vi "Main.vi"(10 "Sub Panel":refnum<vi>, 11 "Module Admin":refnum<class "Delacor_lib_QMH_Module Admin.lvclass">) -> ()   [LabVIEW 2019, in "ANALISIS .lvlib"]
doc: "This template is based off of the Queued Message Handler design pattern and the Queued Message Handler project template that ships with LabVIEW.\n\nThe main difference is that the queue is private to this module and communication between modules is performed via Broadcast and Request events.\n\nRequest events are wrapped in public API methods and are handled in the Event Handling Loop (EHL) of this VI. Any module can register for Broadcast events sent by this module. The EHL generates messages based on user interface actions.\n\nThe Message Handling Loop (MHL) processes messages generated by the EHL, or by other messages. The messages are string values, so new messages can be added easily to the Message Cases case structure in the MHL. Each message cluster can also provide an optional value for Message Data, which is a variant that can be converted to whatever message-specific data is required.\n_____\nBased on Delacor QMH Project Template 5.0.0.82."
uses:
  ANALISIS .lvlib
  <vilib>/Delacor/Delacor QMH/Libraries/Module Admin_class/Delacor_lib_QMH_Module Admin.lvclass
  Module Data--cluster.ctl
  STOP HELPER LOOP ANALISIS Argument--cluster.ctl
  <vilib>/Delacor/Delacor QMH/Libraries/Message Queue_class/Delacor_lib_QMH_Message Queue.lvclass/Delacor_lib_QMH_Message Queue.ctl
  Stop Argument--cluster.ctl
  <vilib>/Delacor/Delacor QMH/Libraries/Module Admin_class/Delacor_lib_QMH_Module Admin.lvclass/Delacor_lib_QMH_Module Admin.ctl
  START HELPER LOOP ANALISIS Argument--cluster.ctl
  acq datos recibir Argument--cluster.ctl
  <vilib>/Utility/miscctls.llb/LVPointTypeDef.ctl
  <vilib>/Delacor/Delacor QMH/Libraries/Message Queue_class/Delacor_lib_QMH_Enqueue Message (Single).vi
  <vilib>/Delacor/Delacor QMH/Libraries/Module Admin_class/Delacor_lib_QMH_Get External Launch.vi
  <vilib>/Utility/error.llb/Error Cluster From Error Code.vi
  <vilib>/ErrorRing/Error Ring.xnode
  <vilib>/Delacor/Delacor QMH/Libraries/Message Queue_class/Delacor_lib_QMH_Message Queue.lvclass
panel:
  out "Bomba encendida":bool
  out "Alarma":bool
  out "Porcentaje del tanque":dbl
  out "Tanque":dbl(slide) scale=0.0..100.0
  out "Estado del tanque":string
  out "Velocidad de bomba de llenado":dbl(knob) scale=0.0..100.0
  out "Velocidad de la bomba de llenado":dbl
  in  "Simulate MHL Error":bool
  in  "Simulate EHL Error":bool
  out "error out":errorcluster
  out "Status":string
  # "Alarmas"
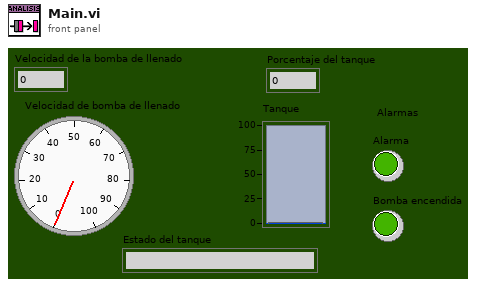
[diagram p1: front panel]
types:
  T1 = typedef "ANALISIS .lvlib/Request Events--cluster.ctl" = cluster{"Stop Module":refnum<user-event>, "Show Panel":refnum<user-event>, "Hide Panel":refnum<user-event>, "Get Module Execution Status":refnum<user-event>, "Show Diagram":refnum<user-event>, "START HELPER LOOP ANALISIS":refnum<user-event>, "STOP HELPER LOOP ANALISIS":refnum<user-event>, "acq datos recibir":refnum<user-event>}
  T2 = typedef "ANALISIS .lvlib/Module Data--cluster.ctl" = cluster{"Status":string}
  T3 = typedef "ANALISIS .lvlib/STOP HELPER LOOP ANALISIS Argument--cluster.ctl" = cluster{"Boolean":bool}
  T4 = enum32{"invalid lock state", "Not Locked", "Locked (No Password)", "Password-protected"}
  T5 = typedef "ANALISIS .lvlib/Stop Argument--cluster.ctl" = cluster{"Origin":string, "Exit via Stop Module Req?":bool, "Wait for Module to stop?":bool}
  T6 = typedef "ANALISIS .lvlib/START HELPER LOOP ANALISIS Argument--cluster.ctl" = cluster{"DELAY TIMEOUT":i32}
  T7 = typedef "ANALISIS .lvlib/acq datos recibir Argument--cluster.ctl" = cluster{"Numeric":dbl}
  T8 = typedef "LVPointTypeDef.ctl" = cluster{"Horizontal":i16, "Vertical":i16}
  T9 = enum32{"Invalid", "Standard", "Closed", "Hidden", "Minimized", "Maximized"}
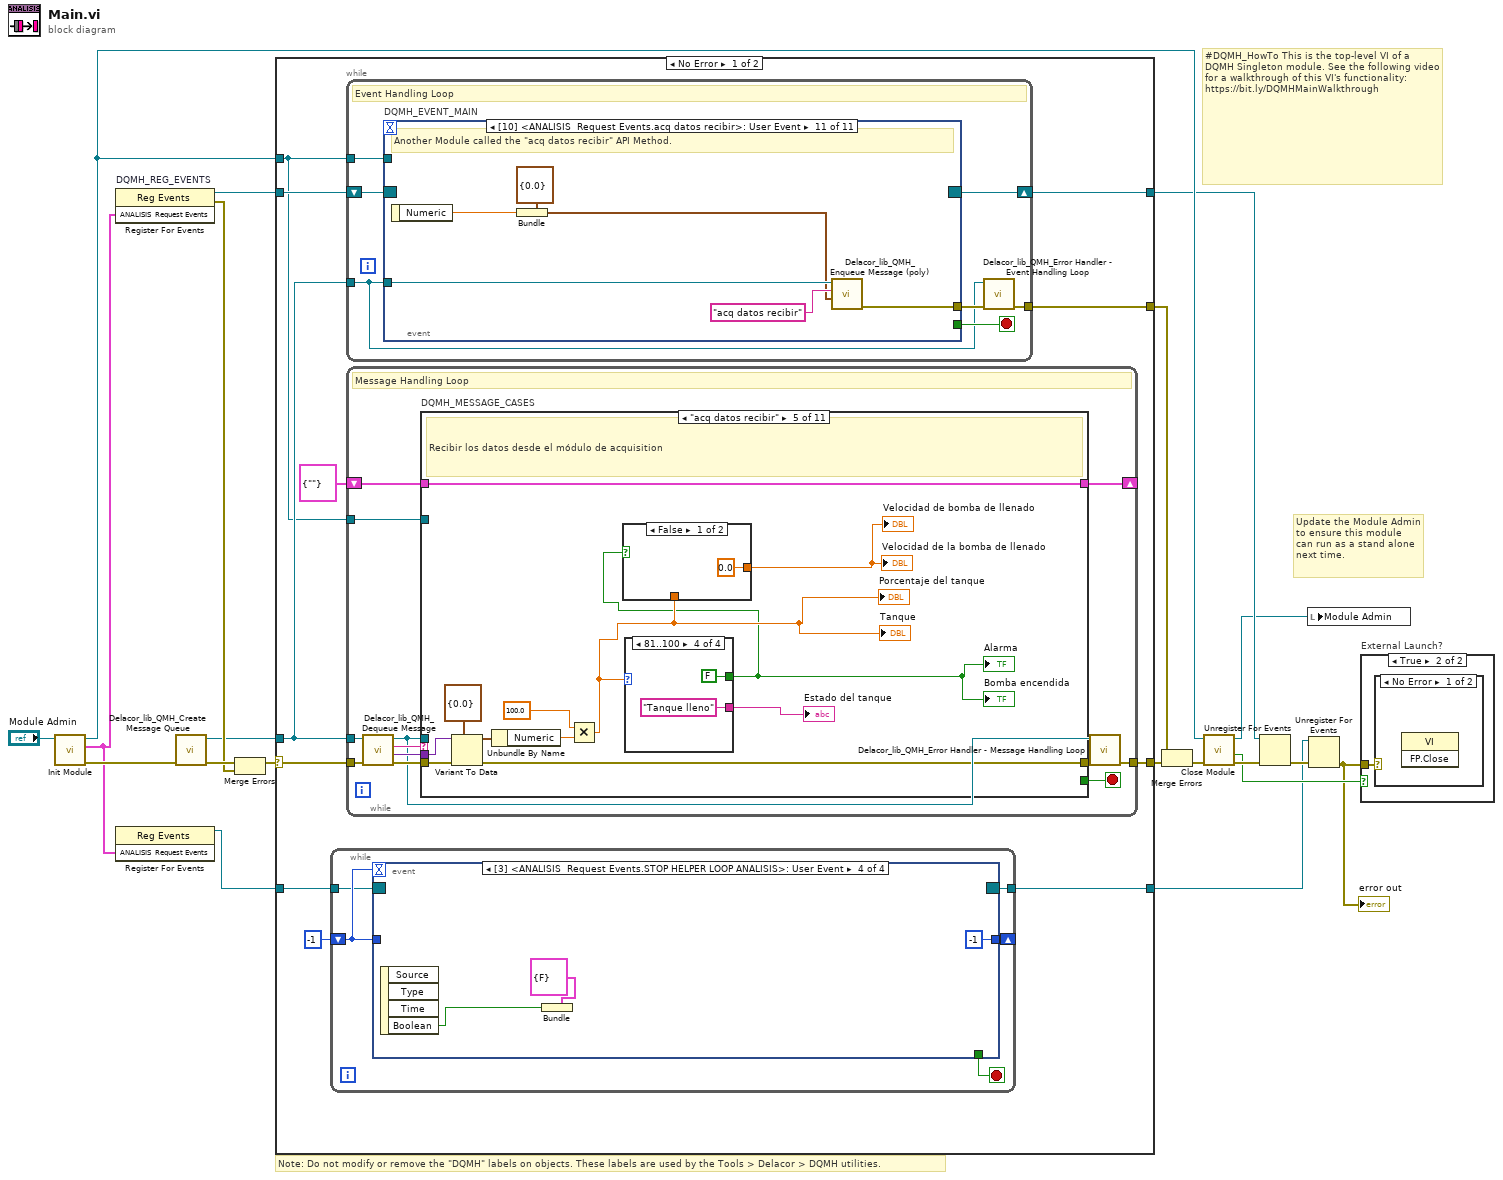
[diagram p0: block diagram]
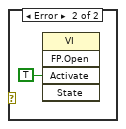
[diagram p3: hidden frame]
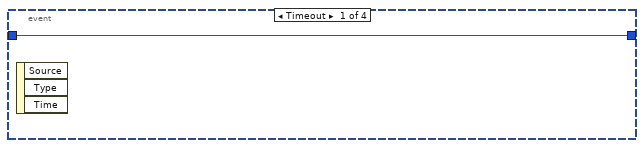
[diagram p4: hidden frame]
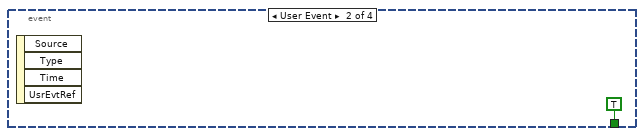
[diagram p5: hidden frame]
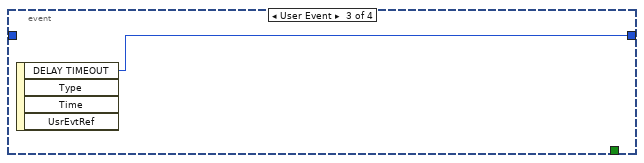
[diagram p6: hidden frame]
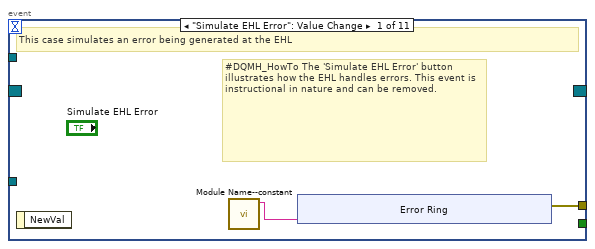
[diagram p7: hidden frame]
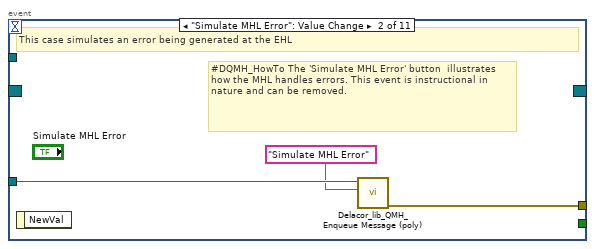
[diagram p8: hidden frame]
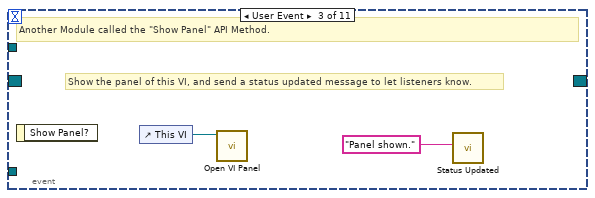
[diagram p9: hidden frame]
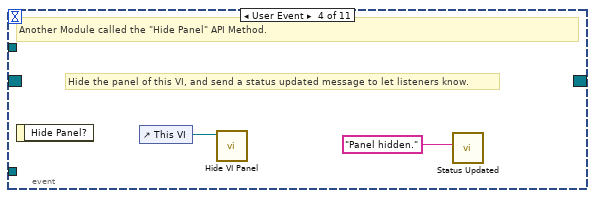
[diagram p10: hidden frame]
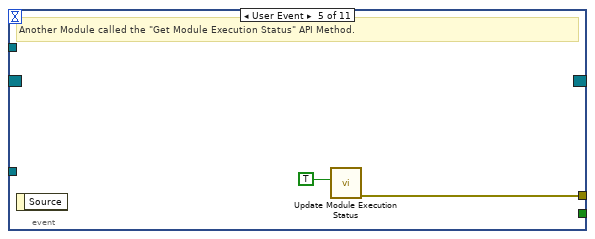
[diagram p11: hidden frame]
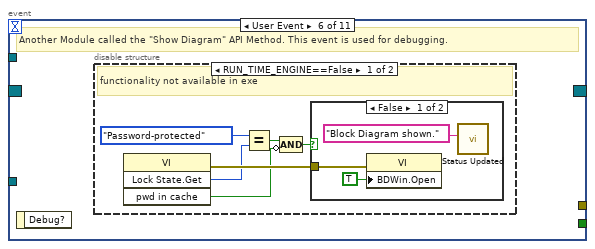
[diagram p12: hidden frame]
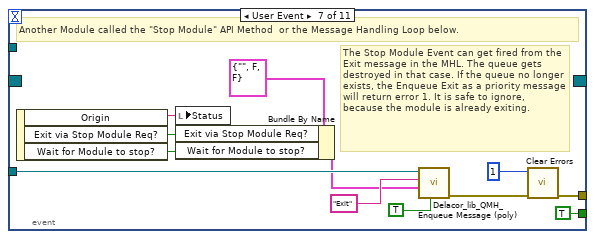
[diagram p15: hidden frame]
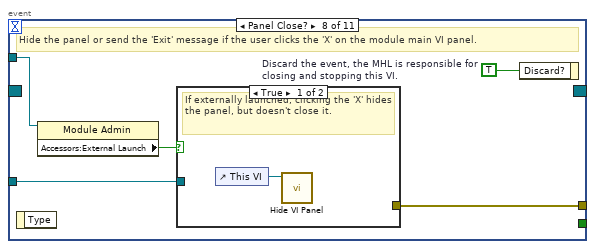
[diagram p16: hidden frame]
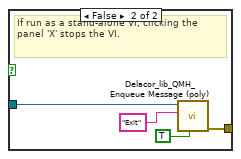
[diagram p17: hidden frame]
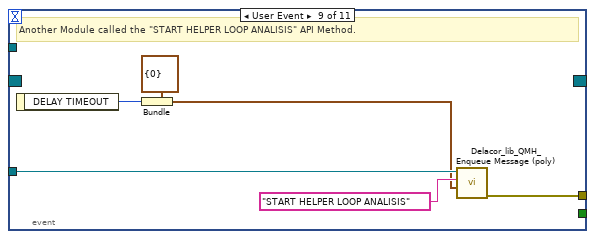
[diagram p18: hidden frame]
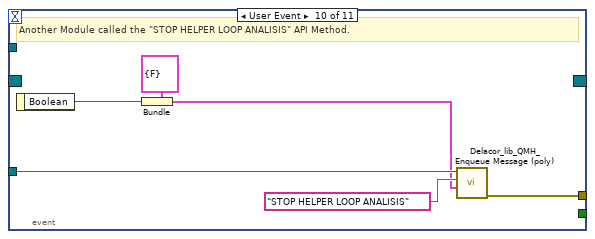
[diagram p19: hidden frame]
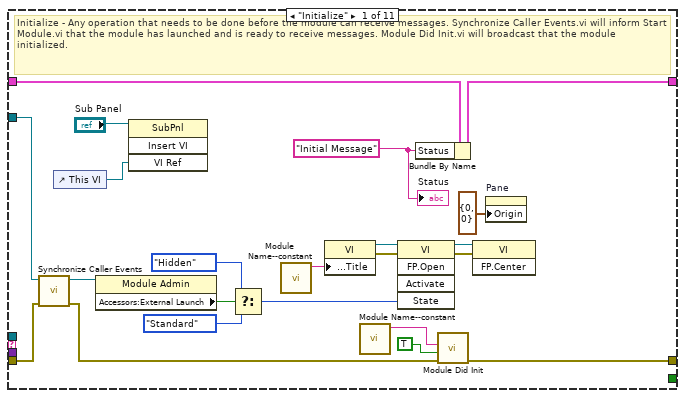
[diagram p20: hidden frame]
diagram:
  # "#DQMH_HowTo This is the top-level VI of a DQMH Singleton module. See the following video for a walkthrough of this VI's functionality: https://bit.ly/DQMHMainWalkthrough"
  # "Note: Do not modify or remove the \"DQMH\" labels on objects. These labels are used by the Tools > Delacor > DQMH utilities."
  # "Update the Module Admin to ensure this module can run as a stand alone next time."
  n1 = call "Init Module.vi"("Singleton Module Admin in"="Module Admin") -> ("error out"=w19:errorcluster, "ANALISIS  Request Events"=w5:T1, "Singleton Module Admin out"=w12:refnum<class "Delacor_lib_QMH_Module Admin.lvclass">)  [unwired: 8 in]
  n2 = register-events "DQMH_REG_EVENTS"(w5) -> (reference out=w10:refnum<event-registration>, error out=w13:errorcluster)  [unwired: 2 in]
  n3 = register-events(w5) -> (reference out=w4:refnum<event-registration>)  [unwired: 2 in, 1 out]
  n4 = call <vilib>:"Delacor_lib_QMH_Create Message Queue.vi"("error in (no error)"=w19) -> ("error out"=w15:errorcluster, "Message Queue"=w9:refnum<class "Delacor_lib_QMH_Message Queue.lvclass">)  [unwired: 9 in]
  n5 = Merge Errors(w15, w13) -> (w14:errorcluster)
  n6 = case shown="No Error" w14 {
    selector: w14 -> [w29 w255]
    tunnel: [w31 w254] -> w20
    tunnel: [w28 w260] -> w11
    tunnel: w10 -> [w26 w260]
    tunnel: w9 -> [w25 w253]
    tunnel: [w30 _] -> w17
    tunnel: w12 -> [w24 w256]
    tunnel: w4 -> [w22 w252]
    tunnel: [w21 w252] -> w2
    frame No Error {
      n7 = while {
        tunnel: [w36] -> w21
        shift-right: [w34] -> _
        shift-left: -1 ("DELAY TIMEOUT") -> [w33]
        tunnel: w22 -> [w32]
        stop <- w35 stop-if-true
        n8 = event shown="[3] <ANALISIS  Request Events.STOP HELPER LOOP ANALISIS>: User Event" {
          selector: w32 -> [_ _ _ _]
          dyn-events: [_ _ _ _] -> w36
          timeout: w33 -> [_ _ _ _]
          tunnel: [_ TRUE ("stop") _ _] -> w35
          tunnel: [w37 _ w39 -1 ("DELAY TIMEOUT")] -> w34
          tunnel: w33 -> [w37 _ _ _]
          event Timeout {
            n9 = event-data() -> ()  [unwired: 1 in, 3 out]
          }
          event User Event {
            n10 = event-data() -> ()  [unwired: 1 in, 4 out]
          }
          event User Event {
            n11 = event-data() -> ("DELAY TIMEOUT"=w39:i32)  [unwired: 1 in, 3 out]
          }
          event User Event {
            n12 = event-data() -> ("Boolean"=w41:bool)  [unwired: 1 in, 3 out]
            n13 = Bundle(cluster=T3 {"Boolean"=FALSE} ("STOP HELPER LOOP ANALISIS Argument"), "Boolean"=w41) -> ()  [unwired: 1 out]
          }
        }
      }
      n14 = while {
        tunnel: w25 -> [w43]
        shift-right: [w46] -> w28
        shift-left: w26 -> [w47]
        tunnel: [w48] -> w30
        tunnel: w24 -> [w44]
        stop <- w45 stop-if-true
        # "Event Handling Loop"
        n15 = event "DQMH_EVENT_MAIN" shown="[10] <ANALISIS  Request Events.acq datos recibir>: User Event" {
          selector: w47 -> [_ _ _ _ _ _ _ _ _ _ _]
          dyn-events: [_ _ _ _ _ _ _ _ _ _ _] -> w46
          timeout: _ -> [_ _ _ _ _ _ _ _ _ _ _]
          tunnel: [_ _ _ _ _ _ TRUE ("Discard?") _ _ _ _] -> w45
          tunnel: w43 -> [_ w60 _ _ _ _ w84 w91 w104 w110 w116]
          tunnel: [w51 w61 _ _ w67 _ w87 w93 w99 w105 w111] -> w49
          tunnel: w44 -> [_ _ _ _ _ _ _ w90 _ _ _]
          event "Simulate EHL Error": Value Change {
            # "#DQMH_HowTo The 'Simulate EHL Error' button  illustrates how the EHL handles errors. This event is instructional in nature and can be removed."
            # "This case simulates an error being generated at the EHL"
            n16 = event-data() -> ()  [unwired: 1 in, 1 out]
            n17 = call "Module Name--constant.vi"() -> ("Module Name"=w50:string)  [unwired: 11 in]
            n18 = xnode "Error Ring"("parameter 0"=w50) -> ("error out"=w51:errorcluster)
          }
          event "Simulate MHL Error": Value Change {
            # "#DQMH_HowTo The 'Simulate MHL Error' button  illustrates how the MHL handles errors. This event is instructional in nature and can be removed."
            # "This case simulates an error being generated at the EHL"
            n19 = event-data() -> ()  [unwired: 1 in, 1 out]
            n20 = call-poly <vilib>:"Delacor_lib_QMH_Enqueue Message (poly).vi"("Message"="Simulate MHL Error", "Message Queue in"=w60) -> ("error out"=w61:errorcluster)  [unwired: 8 in, 1 out]
          }
          event User Event {
            # "Show the panel of this VI, and send a status updated message to let listeners know."
            # "Another Module called the \"Show Panel\" API Method."
            n21 = event-data() -> ()  [unwired: 1 in, 1 out]
            n22 = control-ref of="This VI"() -> (w63:refnum<vi>)
            n23 = call "Open VI Panel.vi"("VI"=w63) -> ()  [unwired: 10 in, 1 out]
            n24 = call "Status Updated.vi"("Status"="Panel shown." ("format string")) -> ()  [unwired: 10 in, 1 out]
          }
          event User Event {
            # "Hide the panel of this VI, and send a status updated message to let listeners know."
            # "Another Module called the \"Hide Panel\" API Method."
            n25 = event-data() -> ()  [unwired: 1 in, 1 out]
            n26 = control-ref of="This VI"() -> (w65:refnum<vi>)
            n27 = call "Hide VI Panel.vi"("VI"=w65) -> ()  [unwired: 10 in, 1 out]
            n28 = call "Status Updated.vi"("Status"="Panel hidden." ("format string")) -> ()  [unwired: 10 in, 1 out]
          }
          event User Event {
            # "Another Module called the \"Get Module Execution Status\" API Method."
            n29 = event-data() -> ()  [unwired: 1 in, 1 out]
            n30 = call "Update Module Execution Status.vi"("Running?"=TRUE) -> ("error out"=w67:errorcluster)  [unwired: 10 in]
          }
          event User Event {
            # "Another Module called the \"Show Diagram\" API Method. This event is used for debugging."
            n31 = event-data() -> ()  [unwired: 1 in, 1 out]
            n32 = disable-structure shown="RUN_TIME_ENGINE==False" {
              frame condition #0 (active) {
                # "functionality not available in exe"
                n33 = invoke class="VI" method="Lock State.Get"() -> (error out=w73:errorcluster, "Get Lock State"=w72:T4, "pwd in cache"=w69:bool)  [unwired: 4 in, 1 out]
                n34 = Equal?(x=T4."Password-protected", y=w72) -> (x = y?=w70:bool)
                n35 = Compound Arithmetic op=AND(w70, invert w69) -> (w68:bool)
                n36 = case shown="False" w68 {
                  tunnel: w73 -> [w76 _]
                  frame False {
                    n37 = property class="VI"(error in=w76, "BDWin.Open"=TRUE ("Block Diagram Window:Open")) -> ()  [unwired: 1 in, 2 out]
                    n38 = call "Status Updated.vi"("Status"="Block Diagram shown." ("format string")) -> ()  [unwired: 10 in, 1 out]
                  }
                  frame True {
                    # "Password-protected VI, and the password is not in the cache. Do not show the diagram."
                  }
                }
              }
              frame condition #1 {
              }
            }
          }
          event User Event {
            # "The Stop Module Event can get fired from the Exit message in the MHL. The queue gets destroyed in that case. If the queue no longer exists, the Enqueue Exit as a priority message will return error 1. It is safe to ignore, because the module is already exiting."
            # "Another Module called the \"Stop Module\" API Method  or the Message Handling Loop below."
            n39 = event-data() -> ("Origin"=w83:string, "Exit via Stop Module Req?"=w79:bool, "Wait for Module to stop?"=w78:bool)  [unwired: 1 in]
            n40 = local write "Status"(w83) -> ()
            n41 = Bundle By Name(cluster=T5 {"Origin"="", "Exit via Stop Module Req?"=FALSE, "Wait for Module to stop?"=FALSE} ("Stop Argument"), "Exit via Stop Module Req?"=w79, "Wait for Module to stop?"=w78) -> (w77:T5)
            n42 = call-poly <vilib>:"Delacor_lib_QMH_Enqueue Message (poly).vi"("Priority Message? (F)"=TRUE, "Message Data"=w77, "Message"="Exit", "Message Queue in"=w84) -> ("error out"=w88:errorcluster)  [unwired: 6 in, 1 out]
            n43 = call <vilib>:"Clear Errors.vi"("error in (no error)"=w88, "specific error code to clear (0: all)"=1) -> ("error out"=w87:errorcluster)  [unwired: 4 in, 1 out]
          }
          event Panel Close? {
            w92 = TRUE  # Discard the event, the MHL is responsible for closing and stopping this VI.
            # "Hide the panel or send the 'Exit' message if the user clicks the 'X' on the module main VI panel."
            n44 = event-data() -> ()  [unwired: 1 in, 1 out]
            n45 = property class="Module Admin"(reference=w90) -> ("Accessors:External Launch"=w89:bool)  [unwired: 1 in, 2 out]
            n46 = case shown="True" w89 {
              tunnel: w91 -> [_ w97]
              tunnel: [_ w98] -> w93
              frame True {
                # "If externally launched, clicking the 'X' hides the panel, but doesn't close it."
                n47 = control-ref of="This VI"() -> (w94:refnum<vi>)
                n48 = call "Hide VI Panel.vi"("VI"=w94) -> ()  [unwired: 10 in, 1 out]
              }
              frame False {
                # "If run as a stand-alone VI, clicking the panel 'X' stops the VI."
                n49 = call-poly <vilib>:"Delacor_lib_QMH_Enqueue Message (poly).vi"("Priority Message? (F)"=TRUE, "Message"="Exit", "Message Queue in"=w97) -> ("error out"=w98:errorcluster)  [unwired: 7 in, 1 out]
              }
            }
            n50 = event-data("Discard?"=w92) -> ()  [unwired: 1 in, 1 out]
          }
          event User Event {
            # "Another Module called the \"START HELPER LOOP ANALISIS\" API Method."
            n51 = event-data() -> ("DELAY TIMEOUT"=w100:i32)  [unwired: 1 in]
            n52 = Bundle(cluster=T6 {"DELAY TIMEOUT"=0} ("START HELPER LOOP ANALISIS Argument"), "DELAY TIMEOUT"=w100) -> (w101:T6)
            n53 = call-poly <vilib>:"Delacor_lib_QMH_Enqueue Message (poly).vi"("Message Data"=w101, "Message"="START HELPER LOOP ANALISIS", "Message Queue in"=w104) -> ("error out"=w99:errorcluster)  [unwired: 7 in, 1 out]
          }
          event User Event {
            # "Another Module called the \"STOP HELPER LOOP ANALISIS\" API Method."
            n54 = event-data() -> ("Boolean"=w106:bool)  [unwired: 1 in]
            n55 = Bundle(cluster=T3 {"Boolean"=FALSE} ("STOP HELPER LOOP ANALISIS Argument"), "Boolean"=w106) -> (w107:T3)
            n56 = call-poly <vilib>:"Delacor_lib_QMH_Enqueue Message (poly).vi"("Message Data"=w107, "Message"="STOP HELPER LOOP ANALISIS", "Message Queue in"=w110) -> ("error out"=w105:errorcluster)  [unwired: 7 in, 1 out]
          }
          event User Event {
            # "Another Module called the \"acq datos recibir\" API Method."
            n57 = event-data() -> ("Numeric"=w112:dbl)  [unwired: 1 in]
            n58 = Bundle(cluster=T7 {"Numeric"=0.0} ("acq datos recibir Argument"), "Numeric"=w112) -> (w113:T7)
            n59 = call-poly <vilib>:"Delacor_lib_QMH_Enqueue Message (poly).vi"("Message Data"=w113, "Message"="acq datos recibir", "Message Queue in"=w116) -> ("error out"=w111:errorcluster)  [unwired: 7 in, 1 out]
          }
        }
        n60 = call-dynamic "Delacor_lib_QMH_Error Handler - Event Handling Loop.vi"("error in (no error)"=w49, "Message Queue in"=w43) -> ("dup error in"=w48:errorcluster)  [unwired: 8 in, 1 out]
      }
      n61 = while {
        tunnel: w25 -> [w119]
        shift-right: [w123] -> _
        shift-left: T2 {"Status"=""} ("Data Cluster") -> [w124]
        tunnel: w29 -> [w127]
        tunnel: [w125] -> w31
        tunnel: w24 -> [w117]
        stop <- w122 stop-if-true
        # "Message Handling Loop"
        n62 = call-dynamic "Delacor_lib_QMH_Dequeue Message.vi"("error in (no error)"=w127, "Message Queue in"=w119) -> ("error out"=w126:errorcluster, "Message Data"=w120:variant, "Message"=w121:string, "Message Queue out"=w118:refnum<class "Delacor_lib_QMH_Message Queue.lvclass">)  [unwired: 6 in]
        n63 = case "DQMH_MESSAGE_CASES" shown="\"acq datos recibir\"" w121 {
          selector: w121 -> [_ _ _ _ _ _ _ _ _ _ w239]
          tunnel: w118 -> [_ _ _ _ _ _ _ _ w209 w231 _]
          tunnel: w126 -> [w148 w152 w158 w164 w176 w191 w193 w198 w216 w237 w241]
          tunnel: [w146 w152 w156 w162 w174 w190 w193 w197 w212 w234 w242] -> w128
          tunnel: w124 -> [w137 w151 w157 w163 w175 w189 w192 w195 w211 w230 w240]
          tunnel: [w136 w151 w157 w163 w175 w189 w192 w195 w211 w230 w240] -> w123
          tunnel: [_ _ _ _ _ _ _ _ _ w229 _] -> w122
          tunnel: w120 -> [_ _ w155 w161 w173 _ _ _ w210 w228 _]
          tunnel: w117 -> [w138 _ _ _ _ _ _ _ w208 w223 _]
          frame "Initialize" {
            w131 = "Initial Message" ("Initial Message")
            # "Initialize - Any operation that needs to be done before the module can receive messages. Synchronize Caller Events.vi will inform Start Module.vi that the module has launched and is ready to receive messages. Module Did Init.vi will broadcast that the module initialized."
            n64 = call "Synchronize Caller Events.vi"("error in (no error)"=w148, "Singleton Module Admin in"=w138) -> ("error out"=w147:errorcluster, "Singleton Module Admin out"=w133:refnum<class "Delacor_lib_QMH_Module Admin.lvclass">)  [unwired: 8 in]
            n65 = control-ref of="This VI"() -> (w129:refnum<vi>)
            n66 = property class="Module Admin"(reference=w133) -> ("Accessors:External Launch"=w142:bool)  [unwired: 1 in, 2 out]
            n67 = invoke class="SubPnl" method="Insert VI"(reference="Sub Panel", "VI Ref"=w129) -> ()  [unwired: 2 in, 4 out]
            n68 = Select(t=T9."Hidden" ("State"), s=w142, f=T9."Standard" ("State")) -> (s? t:f=w139:T9)
            n69 = call "Module Name--constant.vi"() -> ("Module Name"=w145:string)  [unwired: 11 in]
            n70 = property class="VI"("Front Panel.Title"=w145) -> (reference out=w144:refnum<vi>, error out=w150:errorcluster)  [unwired: 2 in]
            n71 = call "Module Name--constant.vi"() -> ("Module Name"=w134:string)  [unwired: 11 in]
            n72 = invoke class="VI" method="FP.Open"(reference=w144, error in=w150, "State"=w139) -> (reference out=w143:refnum<vi>, error out=w149:errorcluster)  [unwired: 2 in, 3 out]
            n73 = Bundle By Name(cluster=w137, "Status"=w131) -> (w136:T2)
            n74 = call "Module Did Init.vi"("error in (no error)"=w147, "Initialized?"=TRUE, "Origin"=w134) -> ("error out"=w146:errorcluster)  [unwired: 8 in]
            n75 = invoke class="VI" method="FP.Center"(reference=w143, error in=w149) -> ()  [unwired: 1 in, 3 out]
            n76 = property on="Pane" class="Pane"("Origin"=T8 {"Horizontal"=0, "Vertical"=0}) -> ()  [unwired: 2 in, 2 out]
            "Status" <- w131
          }
          frame "--- Module Specific ---" {
            # "Separator -- The following cases handle messages specific to this Module."
          }
          frame "START HELPER LOOP ANALISIS" {
            # "#CodeNeeded\n1. Configure this Message Case for handling the \"START HELPER LOOP ANALISIS\" message.\n2. Delete or edit this label when done."
            # "START HELPER LOOP ANALISIS"
            n77 = Variant To Data(error in=w158, type=T6 {"DELAY TIMEOUT"=0} ("START HELPER LOOP ANALISIS Argument"), Variant=w155) -> (data=w153:T6, error out=w156:errorcluster)
            n78 = Unbundle By Name(w153) -> ()  [unwired: 1 out]
          }
          frame "STOP HELPER LOOP ANALISIS" {
            # "#CodeNeeded\n1. Configure this Message Case for handling the \"STOP HELPER LOOP ANALISIS\" message.\n2. Delete or edit this label when done."
            # "STOP HELPER LOOP ANALISIS"
            n79 = Variant To Data(error in=w164, type=T3 {"Boolean"=FALSE} ("STOP HELPER LOOP ANALISIS Argument"), Variant=w161) -> (data=w159:T3, error out=w162:errorcluster)
            n80 = Unbundle By Name(w159) -> ()  [unwired: 1 out]
          }
          frame "acq datos recibir" {
            # "Recibir los datos desde el módulo de acquisition"
            n81 = Variant To Data(error in=w176, type=T7 {"Numeric"=0.0} ("acq datos recibir Argument"), Variant=w173) -> (data=w171:T7, error out=w174:errorcluster)
            n82 = Unbundle By Name(w171) -> ("Numeric"=w170:dbl)
            n83 = Multiply(x=100.0, y=w170) -> (x*y=w167:dbl)
            "Tanque" <- w167
            "Porcentaje del tanque" <- w167
            n84 = case shown="81..100" w167 {
              tunnel: ["Tanque vacío" "Tanque medio" "Tanque alto" "Tanque lleno"] -> w168
              tunnel: [TRUE TRUE TRUE FALSE] -> w165
              frame 1..30, Default {
              }
              frame 31..60 {
              }
              frame 61..80 {
              }
              frame 81..100 {
              }
            }
            "Estado del tanque" <- w168
            "Bomba encendida" <- w165
            "Alarma" <- w165
            n85 = case shown="False" w165 {
              tunnel: w167 -> [_ w180]
              tunnel: [0.0 w178] -> w166
              frame False {
              }
              frame True {
                n86 = Subtract(x=100.0, y=w180) -> (x-y=w178:dbl)
              }
            }
            "Velocidad de la bomba de llenado" <- w166
            "Velocidad de bomba de llenado" <- w166
          }
          frame "---Copy This Frame---" {
            # "Duplicate this frame when creating new messages.  Change this comment in the duplicated frame to describe this message."
            n87 = Merge Errors(w191) -> (w190:errorcluster)
          }
          frame "--- Exit and Error Handling---" {
            # "Separator - The following cases handle errors and exit messages."
          }
          frame "Simulate MHL Error" {
            # "#DQMH_HowTo The 'Simulate MHL Error' button  illustrates how the MHL handles errors. This event is instructional in nature and can be removed."
            # "Simulate an error occurring at the MHL"
            n88 = call "Module Name--constant.vi"() -> ("Module Name"=w194:string)  [unwired: 11 in]
            n89 = xnode "Error Ring"("parameter 0"=w194) -> ("error out"=w196:errorcluster)
            n90 = Merge Errors(w198, w196) -> (w197:errorcluster)
          }
          frame "Error" {
            # "#CodeRecommended - If you ever change the name of this \"Error\" message, you'll need to update the name in the Check Loop Error.vi as well."
            # "#CodeRecommended - If the module is running in standalone mode (External Launch = FALSE), this code will pop up an error dialog and call the 'Exit' message if an error occurs. Add more fine-grained error handling here."
            # "Error - Check the error message data and respond accordingly. This message is sent by the \"Error Handler\" VIs at the end of each loop in this application."
            n91 = property class="Module Admin"(reference=w208) -> ("Accessors:External Launch"=w207:bool)  [unwired: 1 in, 2 out]
            n92 = Variant To Data(error in=w216, type=errorcluster {"status"=FALSE, "code"=0, "source"=""} ("error constant"), Variant=w210) -> (data=w217:errorcluster, error out=w214:errorcluster)
            n93 = call "Module Name--constant.vi"() -> ("Module Name"=w206:string)  [unwired: 11 in]
            n94 = call "Error Reported.vi"("Additional Information"=w206, "Error"=w217) -> ()  [unwired: 9 in, 1 out]
            n95 = case shown="False" w207 {
              tunnel: [w222 _] -> w213
              tunnel: w209 -> [w220 _]
              tunnel: w217 -> [w221 _]
              frame False {
                # "If the module is running standalone, then pop up an error dialog and call the \"Exit\" message."
                n96 = call <vilib>:"Simple Error Handler.vi"("error in (no error)"=w221) -> ()  [unwired: 4 in, 5 out]
                n97 = call-poly <vilib>:"Delacor_lib_QMH_Enqueue Message (poly).vi"("Priority Message? (F)"=TRUE, "Message"="Exit", "Message Queue in"=w220) -> ("error out"=w222:errorcluster)  [unwired: 7 in, 1 out]
              }
              frame True {
                # "If the module was launched externally, calling the Error Reported broadcast VI is the only action performed by the \"Error\" message. The module's caller can then process the error appropriately."
              }
            }
            n98 = Merge Errors(w214, w213) -> (w212:errorcluster)
            n99 = local write "error out"(w212) -> ()
          }
          frame "Exit" {
            w227 = 91  # 91: not all Exit messages will have an argument
            w229 = TRUE  # Stop the VI
            # "Release the message queue reference"
            # "#CodeNeeded - Add any required cleanup code here"
            # "Exit - Exit the application."
            n100 = Variant To Data(error in=w237, type=T5 {"Origin"="", "Exit via Stop Module Req?"=FALSE, "Wait for Module to stop?"=FALSE} ("Stop Argument"), Variant=w228) -> (data=w225:T5, error out=w233:errorcluster)
            n101 = call <vilib>:"Clear Errors.vi"("error in (no error)"=w233, "specific error code to clear (0: all)"=w227) -> ("error out"=w236:errorcluster)  [unwired: 4 in, 1 out]
            n102 = control-ref of="This VI"() -> (w224:refnum<vi>)
            n103 = call-dynamic "Delacor_lib_QMH_Release Message Queue.vi"("error in (no error)"=w236, "Message Queue"=w231) -> ("error out"=w235:errorcluster)  [unwired: 9 in]
            n104 = call "Handle Exit.vi"("Stop Argument"=w225, "Admin in"=w223, "VI reference"=w224) -> ("error out"=w232:errorcluster)  [unwired: 7 in, 1 out]
            n105 = Merge Errors(w235, w232) -> (w234:errorcluster)
          }
          frame Default {
            # "'Default' case only runs if there is a message that isn't defined in any of the other cases.  Output a programming error."
            n106 = call "Module Name--constant.vi"() -> ("Module Name"=w238:string)  [unwired: 11 in]
            n107 = xnode "Error Ring"("parameter 0"=w239, "parameter 1"=w238) -> ("error out"=w243:errorcluster)
            n108 = Merge Errors(w241, w243) -> (w242:errorcluster)
          }
        }
        n109 = call-dynamic "Delacor_lib_QMH_Error Handler - Message Handling Loop.vi"("error in (no error)"=w128, "Message Queue in"=w118) -> ("dup error in"=w125:errorcluster)  [unwired: 8 in, 1 out]
      }
    }
    frame Error {
      # "Synchronize Caller Events.vi will inform Start Module.vi that the module has launched and will let the code calling Start Module.vi register for broadcasts and would permit the caller receive the broadcast that an error occurred at launch time."
      n110 = call-dynamic "Delacor_lib_QMH_Release Message Queue.vi"("error in (no error)"=w255, "Message Queue"=w253) -> ("error out"=w254:errorcluster)  [unwired: 9 in]
      n111 = call "Synchronize Caller Events.vi"("Singleton Module Admin in"=w256) -> ("error out"=w261:errorcluster)  [unwired: 9 in, 1 out]
      n112 = call "Module Name--constant.vi"() -> ("Module Name"=w259:string)  [unwired: 11 in]
      n113 = Format Into String(format string="An error occurred during initialization. %s is no longer running.", w259) -> (resulting string=w257:string)  [unwired: 2 in, 1 out]
      n114 = Merge Errors(w254, w261) -> (w262:errorcluster)
      n115 = call "Error Reported.vi"("Additional Information"=w257, "Error"=w262) -> ()  [unwired: 9 in, 1 out]
    }
  }
  n116 = Merge Errors(w17, w20) -> (w16:errorcluster)
  n117 = call "Close Module.vi"("error in (no error)"=w16, "Module Admin in"=w12) -> ("error out"=w18:errorcluster, "External Launch"=w6:bool, "Module Admin out"=w7:refnum<class "Delacor_lib_QMH_Module Admin.lvclass">)  [unwired: 7 in]
  n118 = Unregister For Events(event registration refnum=w11, error in=w18) -> (error out=w3:errorcluster)
  n119 = local write "Module Admin"(w7) -> ()
  n120 = Unregister For Events(event registration refnum=w2, error in=w3) -> (error out=w1:errorcluster)
  "error out" <- w1
  n121 = case "External Launch?" shown="True" w6 {
    tunnel: w1 -> [_ w263]
    frame False {
    }
    frame True {
      n122 = case shown="No Error" w263 {
        frame No Error {
          n123 = invoke class="VI" method="FP.Close"() -> ()  [unwired: 3 in, 3 out]
        }
        frame Error {
          n124 = invoke class="VI" method="FP.Open"("Activate"=TRUE ("Activate?")) -> ()  [unwired: 4 in, 5 out]
        }
      }
    }
  }
